vi "SaveInstrConfig_LS1.vi"(8 "error in (no error)":errorcluster caption="entrée d'erreur", 11 "Experiment.lvclass":refnum<class "Experiment.lvclass">) -> (0 "error out":errorcluster caption="sortie d'erreur", 3 "Experiment.lvclass 2":refnum<class "Experiment.lvclass">)   [LabVIEW 2010]
uses:
  Experiment Class/Experiment.lvclass
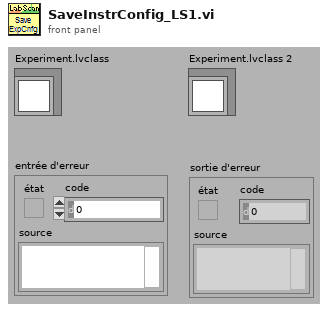
[diagram p1: front panel]
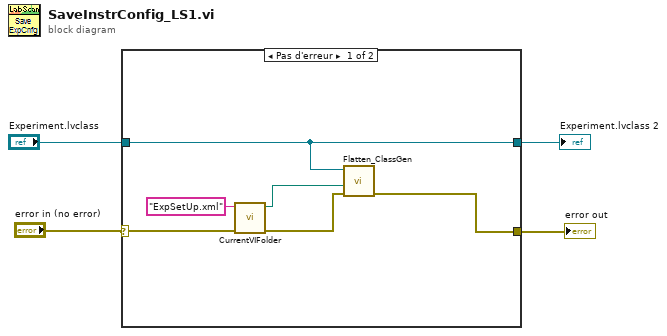
[diagram p0: block diagram]
diagram:
  n1 = case shown="Pas d'erreur" "error in (no error)" {
    selector: "error in (no error)" -> [w6 w12]
    tunnel: "Experiment.lvclass" -> [w5 w11]
    tunnel: [w7 w12] -> w4
    tunnel: [w5 w11] -> w1
    frame No Error {
      n2 = call <userlib>:"CurrentVIFolder.vi"("error in (no error)"=w6, "NomFichier"="ExpSetUp.xml") -> ("error out"=w9:errorcluster, "Chemin"=w8:path)  [unwired: 7 in, 1 out]
      n3 = call <userlib>:"Flatten_ClassGen.vi"("error in (no error)"=w9, "XML File Path"=w8, "Objet LabVIEW"=w5) -> ("error out"=w7:errorcluster)  [unwired: 6 in, 2 out]
    }
    frame Error {
    }
  }
  "error out" <- w4
  "Experiment.lvclass 2" <- w1
